vi "GEOM_GetWCSMod.vi"() -> (2 "response":string)   [LabVIEW 2016]
uses:
  GEOM_VAR_action.ctl
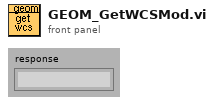
[diagram p1: front panel]
types:
  T1 = typedef "GEOM_VAR_action.ctl" = enum16{"read", "write"}
  T2 = typedef "GEOM_HeaderModule.ctl" = cluster{"name":string, "Keys":string[][]}
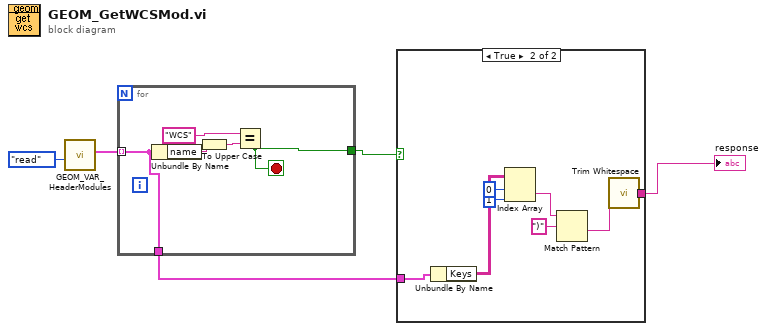
[diagram p0: block diagram]
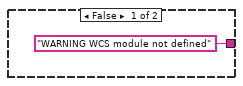
[diagram p2: hidden frame]
diagram:
  n1 = call "GEOM_VAR_HeaderModules.vi"("Action"=GEOM_VAR_action."read") -> ("GEOM_HeaderModules out"=w4:T2[])  [unwired: 1 in, 9 out]
  n2 = for {
    tunnel: w4 -> [w6] mode=indexing
    tunnel: [w7] -> w3
    tunnel: [w6] -> w2
    stop <- w7 stop-if-true
    n3 = Unbundle By Name(w6) -> ("name"=w10:string)
    n4 = To Upper Case(1:w10) -> (0:w8:string)
    n5 = Equal?(x="WCS", y=w8) -> (x = y?=w7:bool)
  }
  n6 = case shown="True" w3 {
    tunnel: w2 -> [_ w19]
    tunnel: ["WARNING WCS module not defined" w12] -> w1
    frame False {
    }
    frame True {
      n7 = Unbundle By Name(w19) -> ("Keys"=w18:string[][])
      n8 = Index Array(array=w18, index (row)=0, index (col)=1 ("disabled index (col)")) -> (element=w15:string)
      n9 = Match Pattern(string=w15, regular expression=")") -> (after substring=w13:string)  [unwired: 4 out]
      n10 = call <vilib>:"Trim Whitespace.vi"("string"=w13) -> ("trimmed string"=w12:string)  [unwired: 1 in]
    }
  }
  "response" <- w1
